vi "CalculateErrorInTopPosition__slk_mt.vi"(3 "add error configure":T2, 7 "position in":T1, 8 "error in (no error)":errorcluster) -> (0 "error out":errorcluster, 5 "position out":T1)   [LabVIEW 2012, in "Lazyboots Menu Tool.lvlib"]
doc: "Gets error in top position."
uses:
  Library/Lazyboots Menu Tool.lvlib
  TypeDef/TypeDef_AddErrorConfigure__slk_mt.ctl
  <vilib>/Utility/miscctls.llb/LVPositionTypeDef.ctl
panel:
  # "CalculateErrorInTopPosition__slk_mt.vi\nGets error in top position.\n\nNOTICE -- YOU MUST LEAVE THIS NOTICE IN PLACE.\n\nCopyright (c) 2011, LIANG LIU Shawn.Liu.cn@gmail.com\nAll rights reserved.\n\nRedistribution and use in source and binary forms, with or without modification, are permitted provided that the following conditions are met:\n-Redistributions of source code must retain the above copyright notice, this list of conditions and the following disclaimer.\n-Redistributions in binary form must reproduce the above copyright notice, this list of conditions and the following disclaimer in the documentation and/or other materials provided with the distribution.\n-Neither the name of the eLp nor the names of its contributors may be used to endorse or promote products derived from this software without specific prior written permission.\n\nTHIS SOFTWARE IS PROVIDED BY THE COPYRIGHT HOLDERS AND CONTRIBUTORS \"AS IS\" AND ANY EXPRESS OR IMPLIED WARRANTIES, INCLUDING, BUT NOT LIMITED TO, THE IMPLIED WARRANTIES OF MERCHANTABILITY AND FITNESS FOR A PARTICULAR PURPOSE ARE DISCLAIMED. IN NO EVENT SHALL THE COPYRIGHT HOLDER OR CONTRIBUTORS BE LIABLE FOR ANY DIRECT, INDIRECT, INCIDENTAL, SPECIAL, EXEMPLARY, OR CONSEQUENTIAL DAMAGES (INCLUDING, BUT NOT LIMITED TO, PROCUREMENT OF SUBSTITUTE GOODS OR SERVICES; LOSS OF USE, DATA, OR PROFITS; OR BUSINESS INTERRUPTION) HOWEVER CAUSED AND ON ANY THEORY OF LIABILITY, WHETHER IN CONTRACT, STRICT LIABILITY, OR TORT (INCLUDING NEGLIGENCE OR OTHERWISE) ARISING IN ANY WAY OUT OF THE USE OF THIS SOFTWARE, EVEN IF ADVISED OF THE POSSIBILITY OF SUCH DAMAGE."
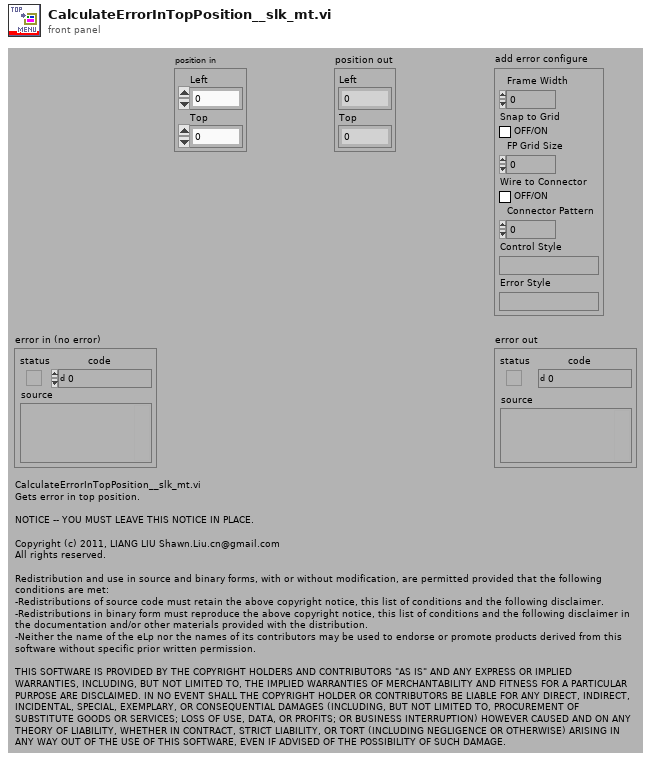
[diagram p1: front panel]
types:
  T1 = typedef "LVPositionTypeDef.ctl" = cluster{"Left":i32, "Top":i32}
  T2 = typedef "Lazyboots Menu Tool.lvlib/TypeDef_AddErrorConfigure__slk_mt.ctl" = cluster{"Frame Width":u32, "Snap to Grid":bool, "FP Grid Size":u32, "Wire to Connector":bool, "Connector Pattern":u32, "Control Style":string, "Error Style":string}
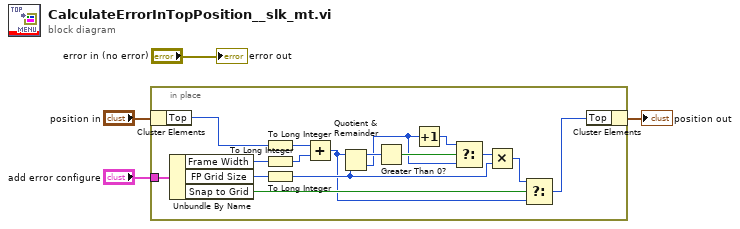
[diagram p0: block diagram]
diagram:
  n1 = in-place {
    in-place-border: "add error configure" -> [w11]
    n2 = in-place-cluster #1("position in") -> ("Top"=w10:i32)
    n3 = Unbundle By Name(w11) -> ("Frame Width"=w13:u32, "FP Grid Size"=w20:u32, "Snap to Grid"=w7:bool)
    n4 = To Long Integer(number=w10) -> (32bit integer=w5:i32)
    n5 = To Long Integer(number=w13) -> (32bit integer=w12:i32)
    n6 = To Long Integer(number=w20) -> (32bit integer=w14:i32)
    n7 = Add(x=w5, y=w12) -> (x+y=w6:i32)
    n8 = Quotient & Remainder(x=w6, y=w14) -> (x-y*floor(x/y)=w19:i32, floor(x/y)=w16:i32)
    n9 = Greater Than 0?(x=w19) -> (x > 0?=w18:bool)
    n10 = Increment(x=w16) -> (x+1=w17:i32)
    n11 = Select(t=w17, s=w18, f=w16) -> (s? t:f=w15:i32)
    n12 = Multiply(x=w15, y=w14) -> (x*y=w9:i32)
    n13 = Select(t=w9, s=w7, f=w6) -> (s? t:f=w8:i32)
    n14 = in-place-cluster #1("Top"=w8) -> (→"position out":T1)
  }
  "error out" <- "error in (no error)"
